vi "Input Stream Control.vi"(0 "input valid":bool, 1 "reset":bool, 5 "start trigger":bool, 7 "burst size":u32, 9 "abort":bool, 11 "fifo timeout":bool, 12 "samples per cycle":u32=1) -> (4 "write stream":bool, 6 "state":T1, 8 "samples processed":u32, 10 "number of overflows":u32, 15 "fifo overflow":bool)   [LabVIEW 2015]
doc: "Controls whether data is written to the DMA FIFO for the acquisition stream. If the burst size is zero, a continuous acquisition is initiated when you set the <B>start trigger</B> parameter to TRUE. If the burst size is greater than zero, the acquisition occurs in bursts of the designated size, and is initiated when the internal state machine is idle and a start trigger is received.\n\nThis VI indicates whether an overflow occurred in the acquisition and also returns the number of overflows that have occurred.\n\nThe internal state machine returns the number of samples processed since the beginning of the most recent acquisition and the current state of the state machine."
uses:
  Stream Control State.ctl
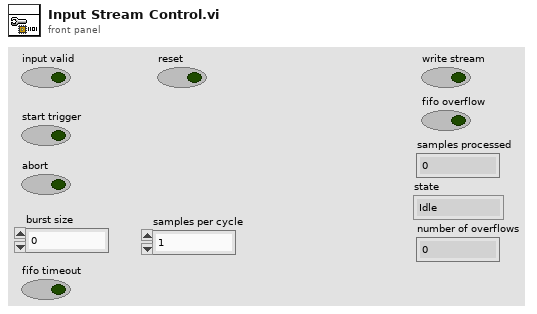
[diagram p1: front panel]
types:
  T1 = typedef "Stream Control State.ctl" = enum16{"Idle", "Active"}
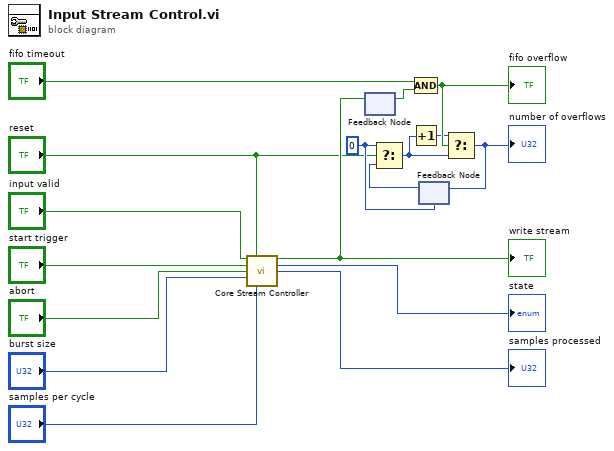
[diagram p0: block diagram]
diagram:
  w4 = u32 0 ("t")
  n1 = call "Core Stream Controller.vi"("input valid"="input valid", "reset"="reset", "start trigger"="start trigger", "abort"="abort", "burst size"="burst size", "samples per cycle"="samples per cycle") -> ("write stream"=w13:bool, "state"=→"state":T1, "samples processed"=→"samples processed":u32)  [unwired: 7 in]
  "write stream" <- w13
  n2 = feedback #1() -> (w15:bool)  [unwired: 1 in]
  n3 = feedback-in #1(w13) -> ()
  n4 = Compound Arithmetic op=AND("fifo timeout", w15) -> (w16:bool)
  "fifo overflow" <- w16
  n5 = feedback #2(w4) -> (w6:u32)
  n6 = Select(t=w4, s="reset", f=w6) -> (s? t:f=w5:u32)
  n7 = Increment(x=w5) -> (x+1=w8:u32)
  n8 = Select(t=w8, s=w16, f=w5) -> (s? t:f=w7:u32)
  "number of overflows" <- w7
  n9 = feedback-in #2(w7) -> ()
